vi "Create Channels for Data Words.vi"(8 "error in (no error)":errorcluster, 10 "Message Param map in":T1(c390), 11 "Iten ref in":T2=18446744073709551615 format="%.0x") -> (0 "error out":errorcluster, 2 "Message Param map out":T1(c390), 3 "Iten ref out":T2=18446744073709551615 format="%.0x")   [LabVIEW 2020, in "Ballard 1553 System Explorer.lvlib"]
uses:
  Ballard 1553 System Explorer.lvlib
  <vilib>/NI VeriStand/Custom Device API/Custom Device API.lvlib
  <vilib>/NI VeriStand/Custom Device API/Custom Device Item Ref.ctl
panel:
  in  "message ID":string
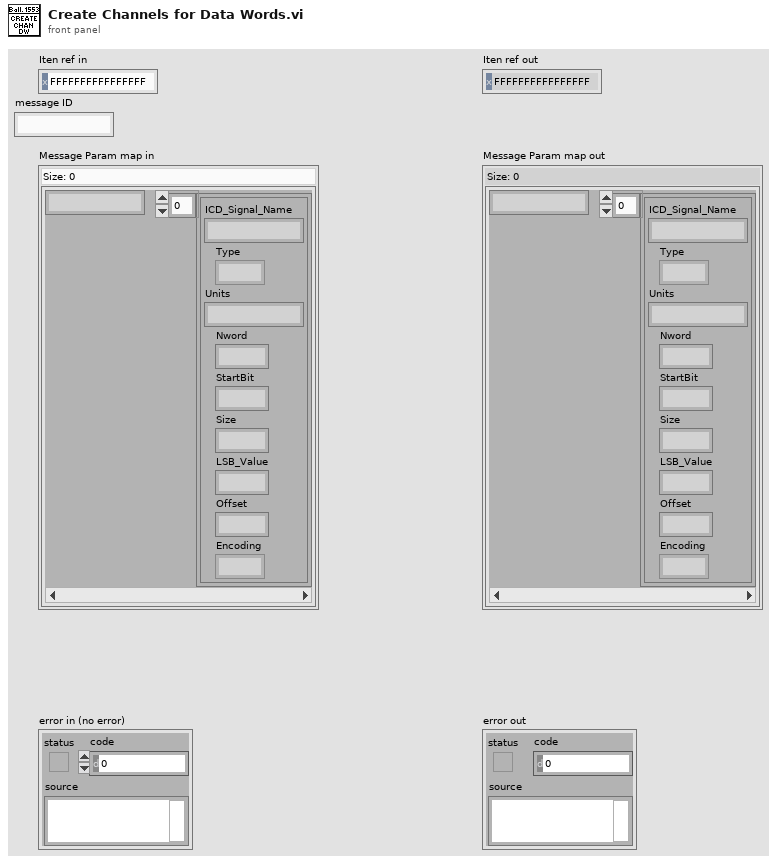
[diagram p1: front panel]
types:
  T1 = map{string, cluster{"ICD_Signal_Name":string, "Type":enum16{"Opaque", "Enum", "Float", "Integer", "Bcd", "Bool"}, "Units":string, "Nword":i32, "StartBit":i32, "Size":i32, "LSB_Value":i32, "Offset":i32, "Encoding":enum16{"None", "2-complement", "Unsigned"}}[]}
  T2 = typedef "Custom Device API.lvlib/Custom Device Item Ref.ctl" = u64
  T3 = cluster{"ICD_Signal_Name":string, "Type":enum16{"Opaque", "Enum", "Float", "Integer", "Bcd", "Bool"}, "Units":string, "Nword":i32, "StartBit":i32, "Size":i32, "LSB_Value":i32, "Offset":i32, "Encoding":enum16{"None", "2-complement", "Unsigned"}}[]
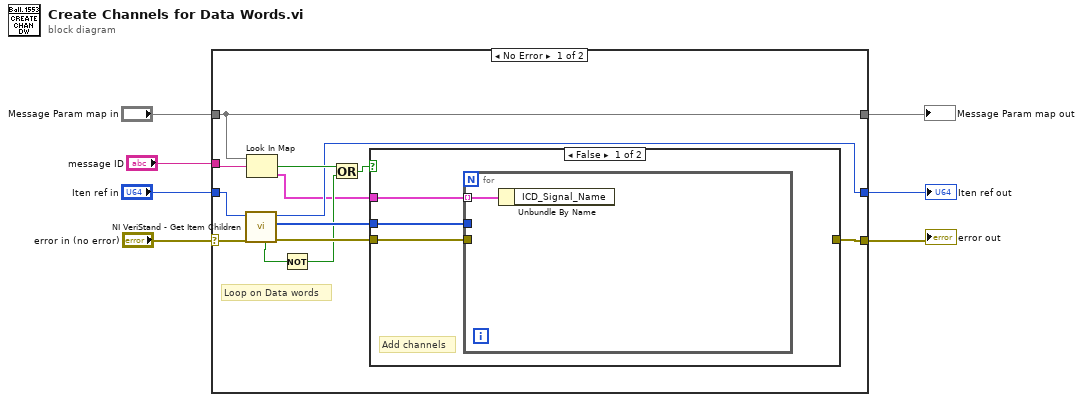
[diagram p0: block diagram]
diagram:
  n1 = case shown="No Error" "error in (no error)" {
    selector: "error in (no error)" -> [w20 w26]
    tunnel: "Iten ref in" -> [w19 w28]
    tunnel: "Message Param map in" -> [w18 w27]
    tunnel: [w9 w28] -> w5
    tunnel: [w18 w27] -> w4
    tunnel: [w15 w26] -> w3
    tunnel: "message ID" -> [w17 _]
    frame No Error {
      # "Loop on Data words"
      n2 = call <vilib>:"NI VeriStand - Get Item Children.vi"("error in (no error)"=w20, "Item Ref in"=w19) -> ("error out"=w14:errorcluster, "Child Refs"=w13:T2[], "Item Ref out"=w9:T2, "Found"=w12:bool)  [unwired: 6 in]
      n3 = Look In Map(map=w18, key=w17) -> (key not found?=w16:bool, value=w8:T3)  [unwired: 1 in]
      n4 = Not(x=w12) -> (.not. x?=w10:bool)
      n5 = Or(x=w16, y=w10) -> (x .or. y?=w11:bool)
      n6 = case shown="False" w11 {
        tunnel: [_ w25] -> w15
        tunnel: w14 -> [w23 w25]
        tunnel: w13 -> [w22 _]
        tunnel: w8 -> [w21 _]
        frame False {
          # "Add channels"
          n7 = for {
            tunnel: w23 -> [_]
            tunnel: w22 -> [_]
            tunnel: w21 -> [w24] mode=indexing
            n8 = Unbundle By Name(w24) -> ()  [unwired: 1 out]
          }
        }
        frame True {
          # "No key or no DW, do nothing"
        }
      }
    }
    frame Error {
    }
  }
  "error out" <- w3
  "Iten ref out" <- w5
  "Message Param map out" <- w4
